vi "Write Parent Fully Qualified Name.vi"(10 "Parent Fully Qualified Name":string, 11 "UniqueName in":refnum<class "UniqueName.lvclass">) -> (3 "UniqueName out":refnum<class "UniqueName.lvclass">)   [LabVIEW 2013, in "UniqueName.lvlib" / "UniqueName.lvclass"]
uses:
  UniqueName.lvclass
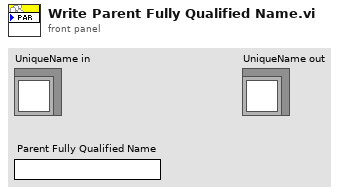
[diagram p1: front panel]
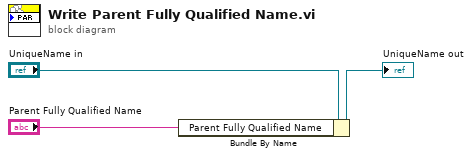
[diagram p0: block diagram]
diagram:
  n1 = Bundle By Name(cluster="UniqueName in", "Parent Fully Qualified Name"="Parent Fully Qualified Name") -> (→"UniqueName out":refnum<class "UniqueName.lvclass">)
